vi "Get Service Class Instances.vi"() -> (3 "service instances":refnum<class "ServiceBase.lvclass">[](array[class]))   [LabVIEW 2019, in "Generated_server.lvlib"]
uses:
  Generated_server.lvlib
  RPC Service/Session/Session.lvclass
  <vilib>/gRPC/LabVIEW gRPC Servicer/ServiceBase/ServiceBase.lvclass
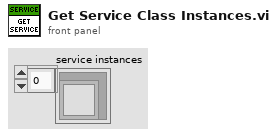
[diagram p1: front panel]
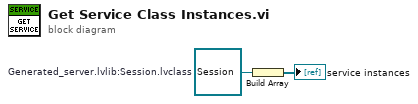
[diagram p0: block diagram]
diagram:
  w1 = refnum<class "Session.lvclass"> refnum  # Generated_server.lvlib:Session.lvclass
  n1 = Build Array(w1) -> (→"service instances":refnum<class "Session.lvclass">[])
